vi "simx Get Integer Signal.vi"(7 "operationMode":i32, 8 "error in (no error)":errorcluster, 9 "signalValue":i32, 10 "signalName":string, 11 "clientID":i32) -> (0 "error out":errorcluster, 1 "signalValue out":i32, 3 "function return":i32)   [LabVIEW 2019, in "PXL_V-REP.lvlib"]
doc: "EXTAPI_DLLEXPORT simxInt simxGetIntegerSignal(simxInt clientID,const simxChar* signalName,simxInt* signalValue,simxInt operationMode);"
uses:
  PXL_V-REP.lvlib
  <userlib>/V-REP/remoteApi.dll
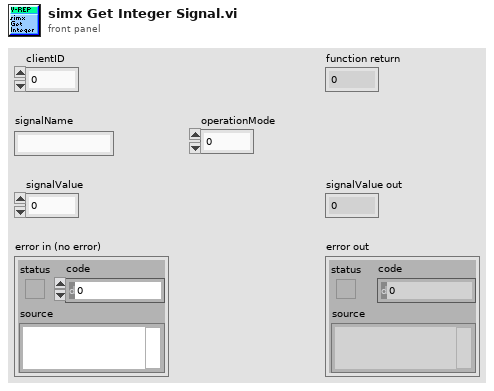
[diagram p1: front panel]
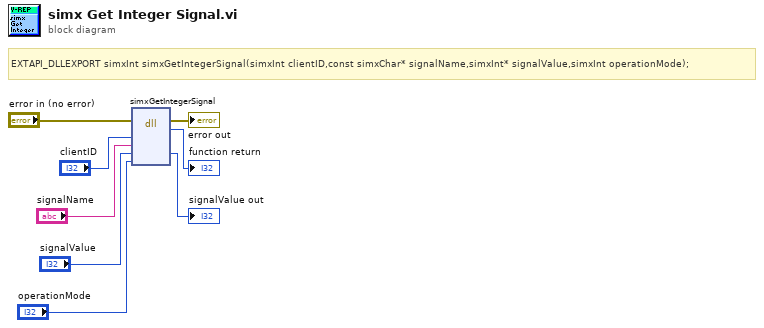
[diagram p0: block diagram]
diagram:
  # "EXTAPI_DLLEXPORT simxInt simxGetIntegerSignal(simxInt clientID,const simxChar* signalName,simxInt* signalValue,simxInt operationMode);"
  n1 = dll-call lib="C:/Program Files (x86)/National Instruments/LabVIEW 2019/user.lib/V-REP/remoteApi.*" fn="simxGetIntegerSignal"(error in="error in (no error)", "clientID"="clientID", "signalName"="signalName", "signalValue"="signalValue", "operationMode"="operationMode") -> (error out=→"error out":errorcluster, →"function return":i32, "signalValue"=→"signalValue out":i32)  [unwired: 5 in, 1 out]
